vi "DB - [AMS].[Execute].[Message].vi"(0 "connection reference":T3, 1 "DB Connection":T4={"Open"=TRUE, "Close"=TRUE}, 2 "<TOP>":string, 3 "DB - [AMS].[Execute].[Message] Enum":T1, 5 "AMS Execute Message ColNames":T2[](array[typedef])=[enum."[MessageNo]", enum."[SoftwareSolutionId]", enum."[SoftwareSolutionName]", enum."[PlantId]", enum."[MessageLogNo]", enum."[ReceivedOn]", enum."[MessageCode]", enum."[ShortDescription]", enum."[Message]", enum."[SmsMessage]", enum."[TransactionNo]", enum."[TransactionRunNo]", enum."[MessageInitiator]", enum."[Remarks]", enum."[MsgCreatedOn]", enum."[IsToSendSms]", enum."[IsToSendEmail]", enum."[SmsContent]", enum."[EmailContent]", enum."[MobileNos]", enum."[EmailAddresses]"], 9 "<Data> (0xFFFE autodetect)":string[](array[string]), 11 "error in (no error)":errorcluster, 12 "<SIGN>":string, 13 "[MessageNo]":string, 14 "<CONDITIONS>":string) -> (4 "connection reference":T3, 6 "2D data":string[][](array[string]), 10 "SQL Statement":string, 15 "SUMMARY":errorcluster)   [LabVIEW 2013]
uses:
  <vilib>/addons/database/Connection.llb/Conn ObjectReference.ctl
  Controls/DB - OpenClose.ctl
  Controls/DB - [AMS].[Execute].[Message] ColNames.ctl
  Controls/DB - [AMS].[Execute].[Message] Enum.ctl
  Controls/Global AMS.vi
  Controls/Global SRTRS.vi
  <vilib>/addons/database/Connection.llb/DB Tools Open Connec (String).vi
  <vilib>/addons/database/Connection.llb/Conn Execute.vi
  <vilib>/addons/database/Recordset.llb/Rec Fetch Recordset Data (R).vi
  <vilib>/addons/database/Recordset.llb/Rec Destroy - Connection.vi
  <vilib>/addons/database/_DB Variant To Data/Database Variant To Data.xnode
  <vilib>/addons/database/NI_Database_API.lvlib
panel:
  out "Close":errorcluster
  in  "AMS.Execute.MESSAGE (IMPT to leave it in CAPS)":string="AMS.Execute.MESSAGE"
  out "Connection Information":T5={"Connection "="SQL Server 32bit HPEnvy", "Username"="admin", "Password"="admin123"}
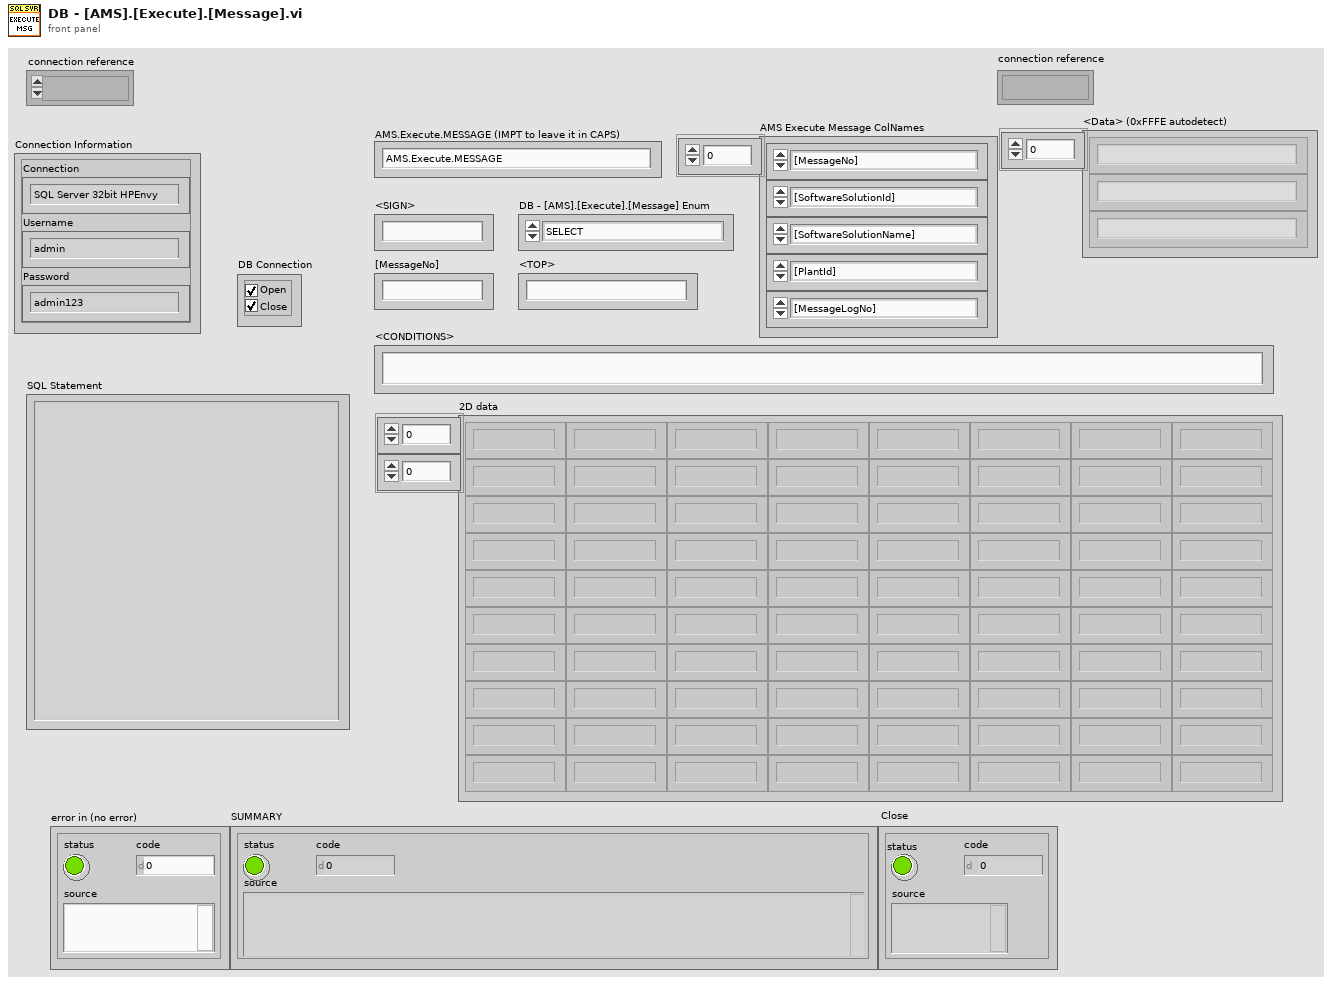
[diagram p1: front panel]
types:
  T1 = typedef "DB - [AMS].[Execute].[Message] Enum.ctl" = enum16{"SELECT", "SELECT (Multi-Conditions)", "UPDATE", "RE-INSERT"}
  T2 = typedef "DB - [AMS].[Execute].[Message] ColNames.ctl" = enum16{"[MessageNo]", "[LanguageId]", "[SoftwareSolutionId]", "[SoftwareSolutionName]", "[PlantId]", "[SystemId]", "[StationId]", "[MessageLogNo]", "[ReceivedOn]", "[MessageCode]", "[ShortDescription]", "[Message]", "[SmsMessage]", "[SuppMessage1]", "[SuppMessage2]", "[SuppMessage3]", "[TransactionNo]", "[TransactionRunNo]", "[MessageInitiator]", "[Remarks]", "[MsgCreatedOn]", "[IsToSendSms]", "[IsToSendEmail]", "[IsToSendCommMedium1]", "[IsToSendCommMedium2]", "[SmsContent]", "[EmailContent]", "[CommMed1Content]", "[CommMed2Content]", "[MobileNos]", "[EmailAddresses]", "[CommMedium1Ids]", "[CommMedium2Ids]", "[LastAttemptedCommMed]", "[LastAttemptedNo]", "[LastAttemptedOn]", "[IsSmsSent]", "[IsEmailSent]", "[IsCommMedium1Sent]", "[IsCommMedium2Sent]", "[OverallSentStatus]", "[StatusUpdatedOn]", "[IsArchived]"}
  T3 = typedef "NI_Database_API.lvlib/Conn ObjectReference.ctl" = refnum<k1>
  T4 = typedef "DB - OpenClose.ctl" = cluster{"Open":bool, "Close":bool}
  T5 = cluster{"Connection ":string, "Username":string, "Password":string}
  T6 = typedef "Enum - InteractiveMode-SubVIMode.ctl" = enum16{"Interactive", "subVI Mode"}
  T7 = typedef "Connection Information Cluster.ctl" = cluster{"Connection ":string, "Username":string, "Password":string}
  T8 = typedef "DB - DB.Schema.Table.ctl" = cluster{"DB":string, "Schema":string, "Table":string}
  T9 = typedef "NI_Database_API.lvlib/Rec ObjectReference.ctl" = refnum<k1>
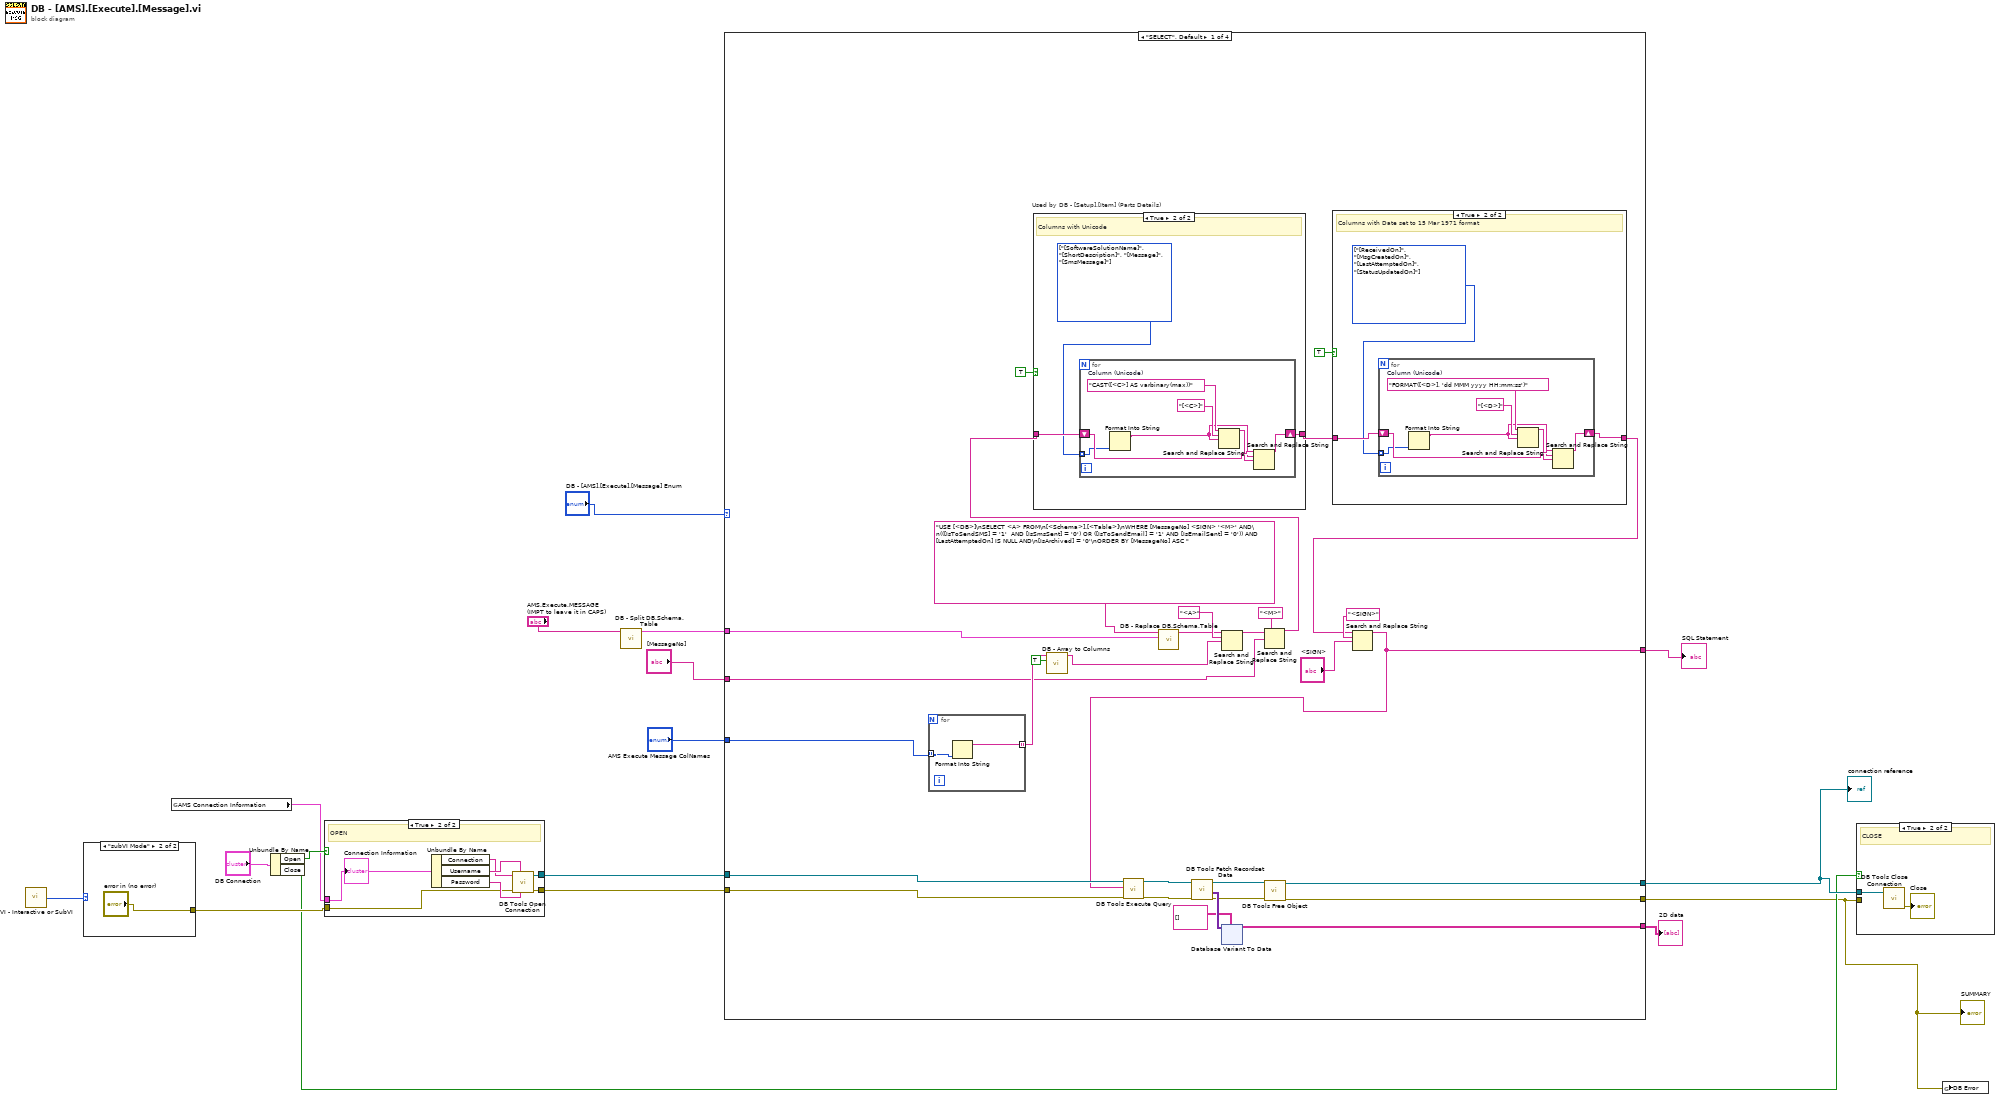
[diagram p0: block diagram]
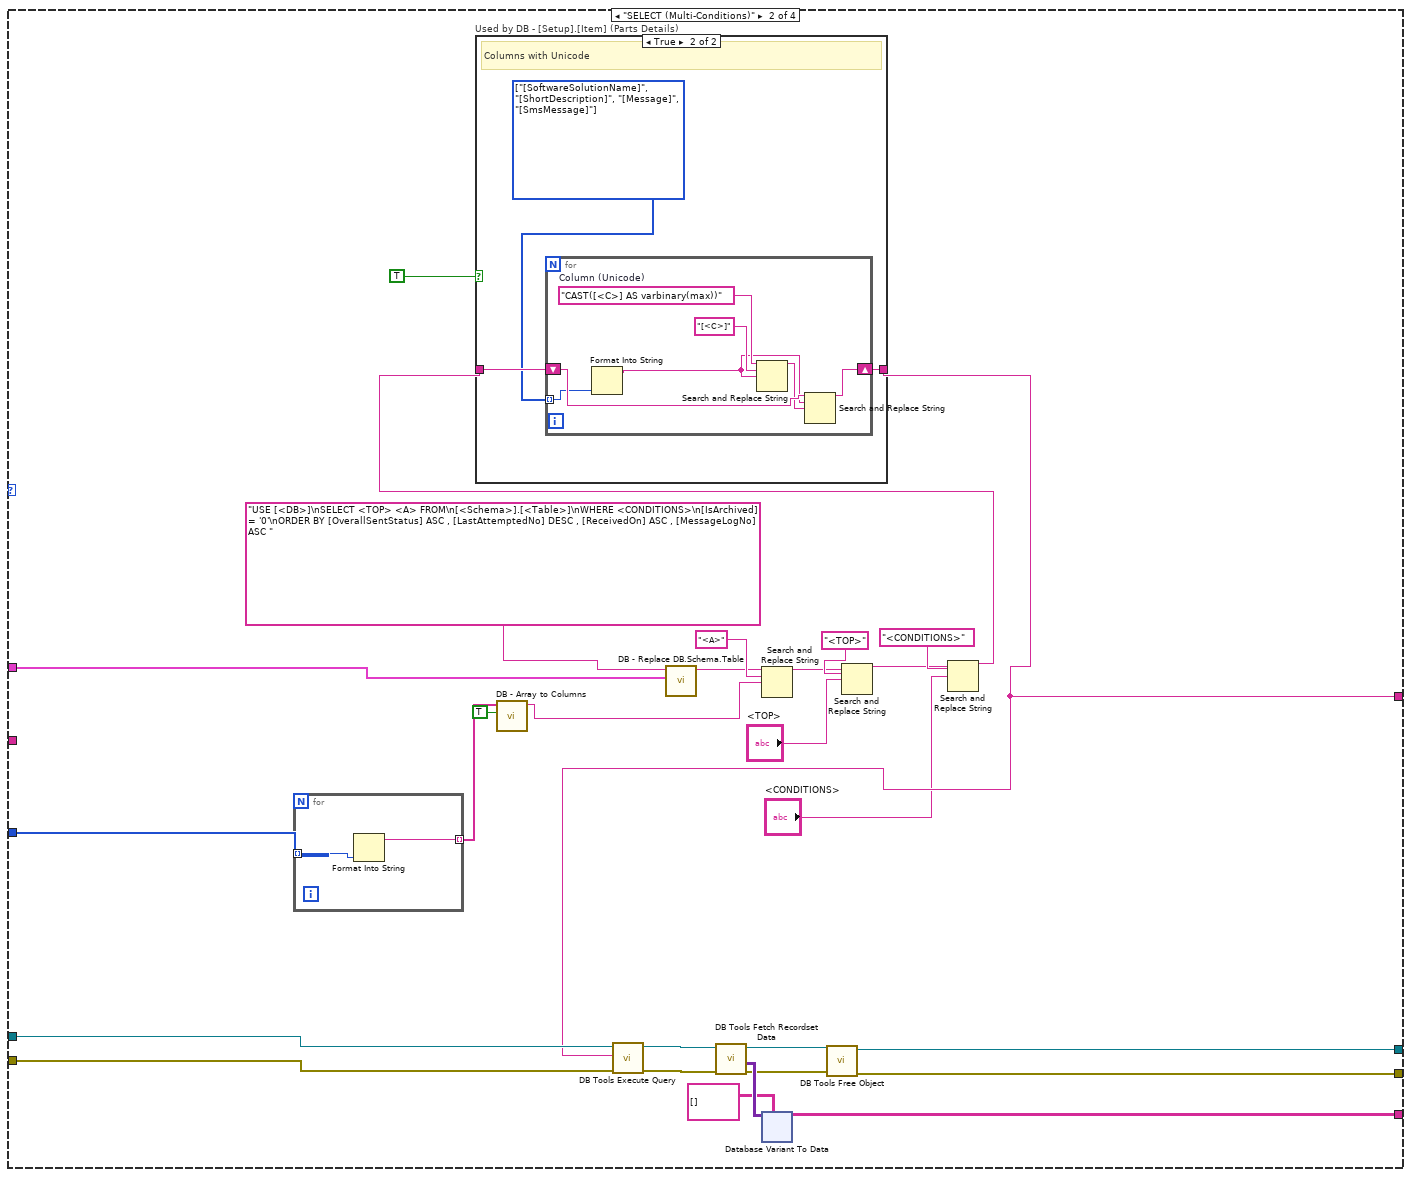
[diagram p4: hidden frame]
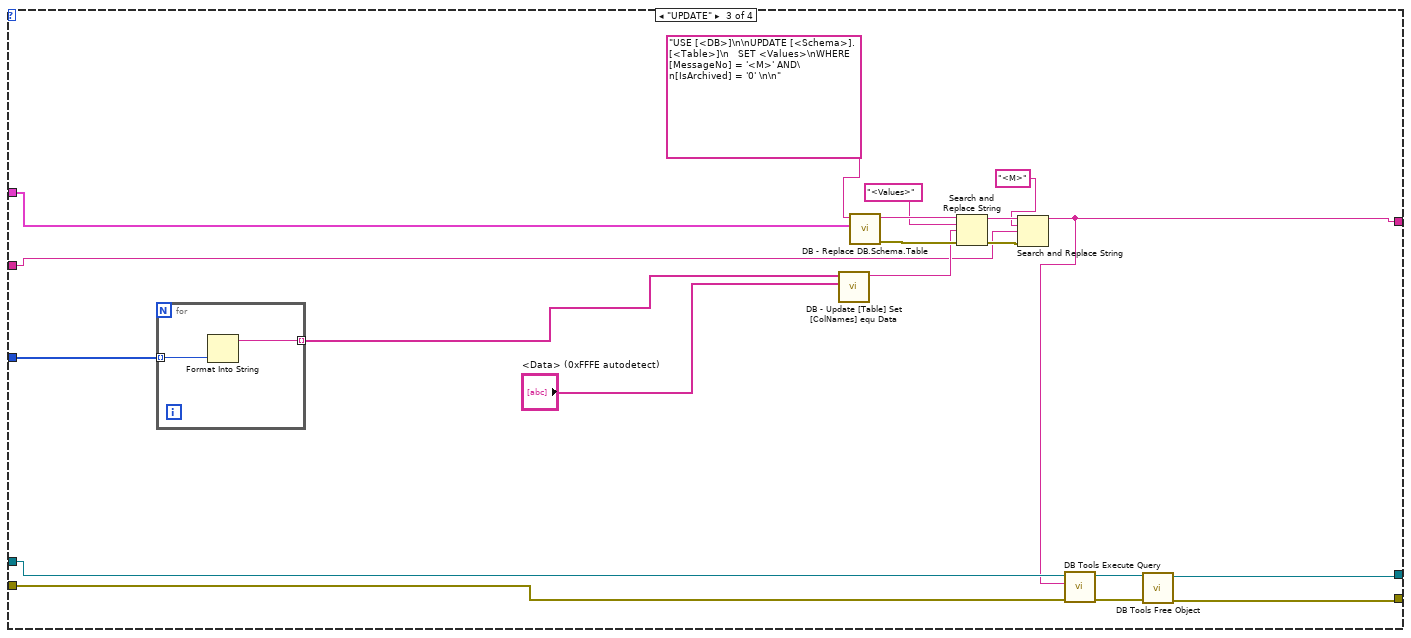
[diagram p6: hidden frame]
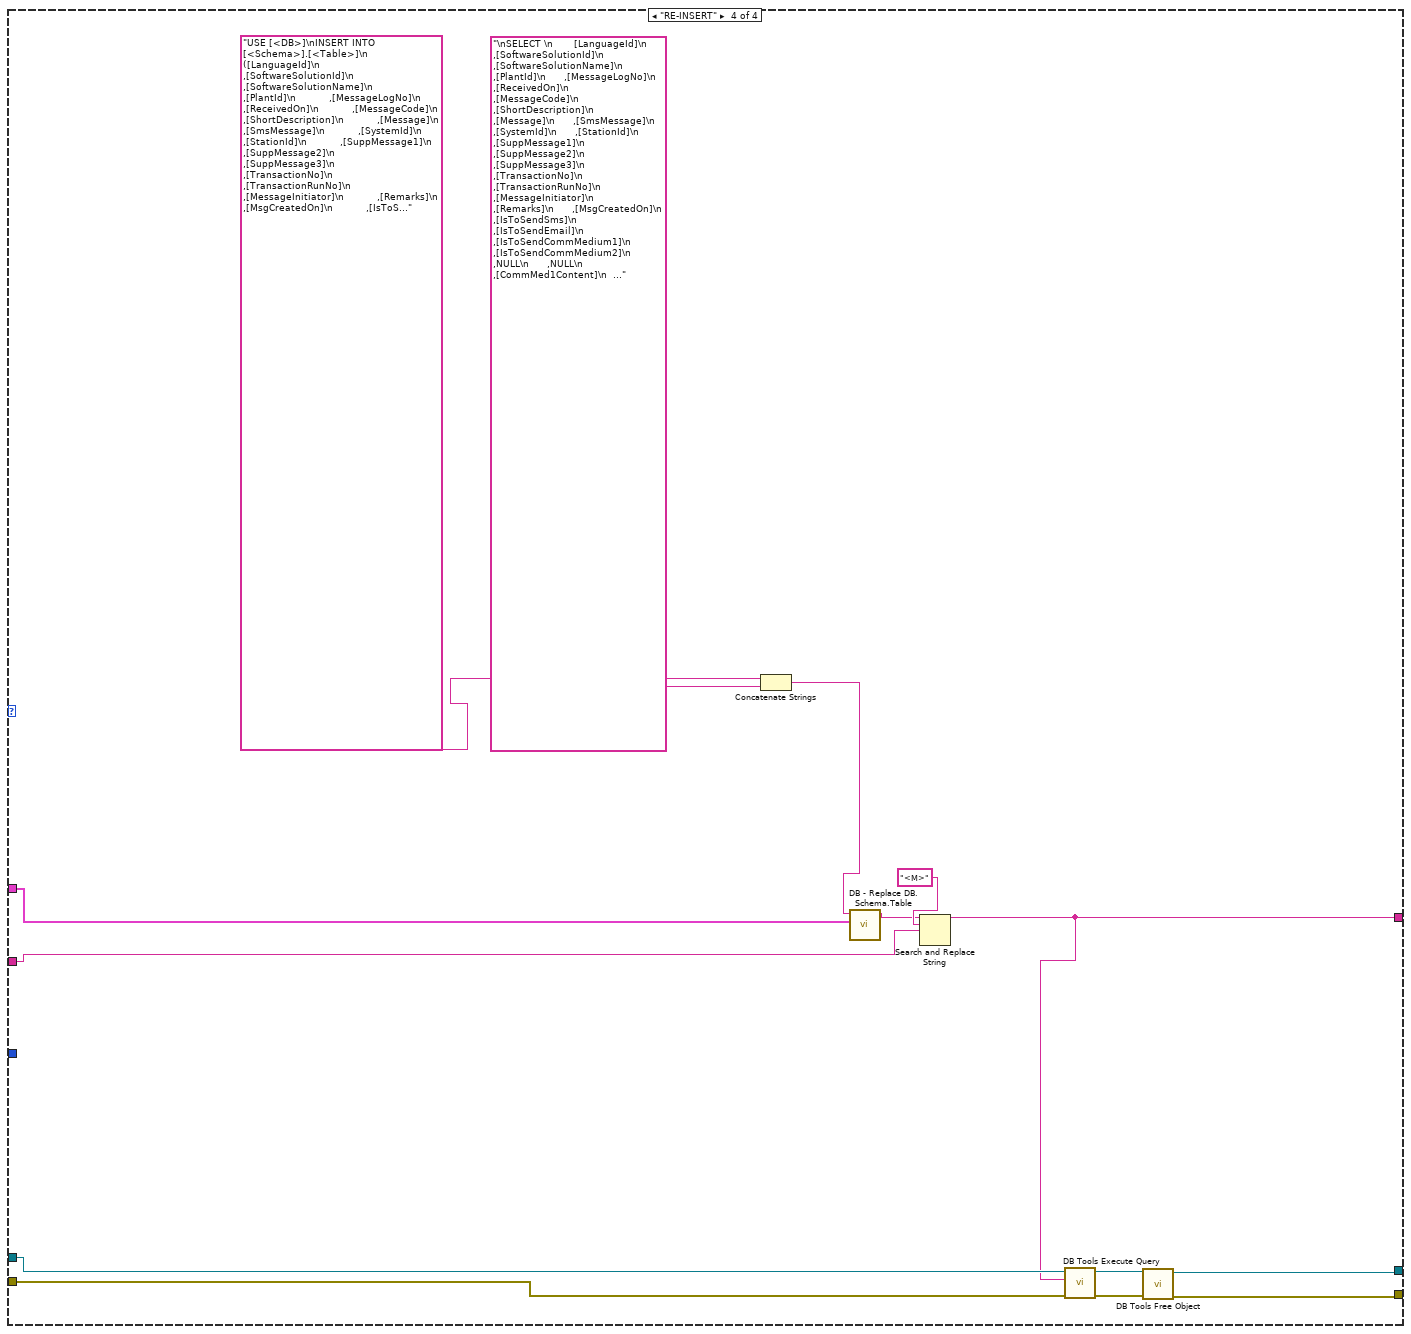
[diagram p7: hidden frame]
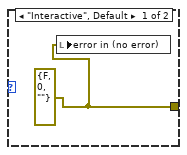
[diagram p9: hidden frame]
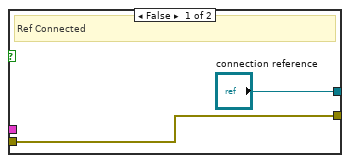
[diagram p10: hidden frame]
diagram:
  n1 = call "VI - Interactive or SubVI.vi"() -> ("Mode"=w15:T6)  [unwired: 5 in]
  n2 = case shown="\"subVI Mode\"" w15 {
    tunnel: [w18 "error in (no error)"] -> w14
    frame "Interactive", Default {
      w18 = errorcluster {"status"=FALSE, "code"=0, "source"=""} ("error in (no error)")
      n3 = local write "error in (no error)"(w18) -> ()
    }
    frame "subVI Mode" {
    }
  }
  n4 = global read "Global AMS.vi" "AMS Connection Information"() -> (w6:T7)
  n5 = Unbundle By Name("DB Connection") -> ("Open"=w16:bool, "Close"=w10:bool)
  n6 = case shown="True" w16 {
    tunnel: ["connection reference" w25] -> w13
    tunnel: w14 -> [w20 w24]
    tunnel: [w20 w23] -> w12
    tunnel: w6 -> [_ w22]
    frame False {
      # "Ref Connected"
    }
    frame True {
      # "OPEN"
      n7 = Unbundle By Name(w22) -> ("Connection"=w27:string, "Username"=w28:string, "Password"=w26:string)
      n8 = call-poly <vilib>:"DB Tools Open Connection.vi"("password"=w26, "userID"=w28, "error in (no error)"=w24, "connection information"=w27) -> ("error out"=w23:errorcluster, "connection reference"=w25:T3)  [unwired: 4 in]
      "Connection Information" <- w22
    }
  }
  n9 = call "DB - Split DB.Schema.Table.vi"("DB.Schema.Table"="AMS.Execute.MESSAGE (IMPT to leave it in CAPS)") -> ("DB.Schema.Table"=w9:T8)  [unwired: 10 in]
  n10 = case shown="\"SELECT\", Default" "DB - [AMS].[Execute].[Message] Enum" {
    tunnel: w13 -> [w52 w148 w215 w239]
    tunnel: w12 -> [w51 w147 w216 w240]
    tunnel: [w50 w146 w218 w242] -> w11
    tunnel: w9 -> [w49 w145 w224 w246]
    tunnel: [w47 w143 w217 w241] -> w8
    tunnel: "AMS Execute Message ColNames" -> [w44 w141 w213 _]
    tunnel: "[MessageNo]" -> [w39 _ w222 w245]
    tunnel: [w36 w133 w214 w238] -> w3
    tunnel: [w32 w132 _ _] -> w1
    frame "SELECT", Default {
      n11 = for {
        tunnel: w44 -> [w82] mode=indexing
        tunnel: [w81] -> w43 mode=indexing
        n12 = Format Into String(w82) -> (resulting string=w81:string)  [unwired: 3 in, 1 out]
      }
      n13 = call "DB - Array to Columns.vi"("Exclude []"=TRUE, "Array"=w43) -> ("[Columns]"=w38:string)  [unwired: 9 in]
      n14 = call "DB - Replace DB.Schema.Table.vi"("DB.Schema.Table"=w49, "string in"="USE [<DB>]\nSELECT <A> FROM\n[<Schema>].[<Table>]\nWHERE [MessageNo] <SIGN> '<M>' AND\n(([IsToSendSMS] = '1'  AND [IsSmsSent] = '0') OR ([IsToSendEmail] = '1' AND [IsEmailSent] = '0')) AND [LastAttemptedOn] IS NULL AND\n[IsArchived] = '0'\nORDER BY [MessageNo] ASC ") -> ("string out"=w33:string)  [unwired: 8 in, 1 out]
      n15 = Search and Replace String(input string=w33, search string="<A>", replace string=w38) -> (result string=w46:string)  [unwired: 5 in, 3 out]
      n16 = Search and Replace String(input string=w46, search string="<M>", replace string=w39) -> (result string=w42:string)  [unwired: 5 in, 3 out]
      n17 = case "Used by DB - [Setup].[Item] (Parts Details)" shown="True" TRUE {
        tunnel: w42 -> [w70 w73]
        tunnel: [w70 w72] -> w30
        frame False {
        }
        frame True {
          w71 = T2[] [enum."[SoftwareSolutionName]", enum."[ShortDescription]", enum."[Message]", enum."[SmsMessage]"] items=["[MessageNo]", "[LanguageId]", "[SoftwareSolutionId]", "[SoftwareSolutionName]", "[PlantId]", "[SystemId]", "[StationId]", "[MessageLogNo]", "[ReceivedOn]", "[MessageCode]", "[ShortDescription]", "[Message]", "[SmsMessage]", "[SuppMessage1]", "[SuppMessage2]", "[SuppMessage3]", "[TransactionNo]", "[TransactionRunNo]", "[MessageInitiator]", "[Remarks]", "[MsgCreatedOn]", "[IsToSendSms]", "[IsToSendEmail]", "[IsToSendCommMedium1]", "[IsToSendCommMedium2]", "[SmsContent]", "[EmailContent]", "[CommMed1Content]", "[CommMed2Content]", "[MobileNos]", "[EmailAddresses]", "[CommMedium1Ids]", "[CommMedium2Ids]", "[LastAttemptedCommMed]", "[LastAttemptedNo]", "[LastAttemptedOn]", "[IsSmsSent]", "[IsEmailSent]", "[IsCommMedium1Sent]", "[IsCommMedium2Sent]", "[OverallSentStatus]", "[StatusUpdatedOn]", "[IsArchived]"]
          # "Columns with Unicode"
          n18 = for {
            shift-right: [w76] -> w72
            shift-left: w73 -> [w80]
            tunnel: w71 -> [w75] mode=indexing
            w79 = "CAST([<C>] AS varbinary(max))"  # Column (Unicode)
            n19 = Format Into String(w75) -> (resulting string=w74:string)  [unwired: 3 in, 1 out]
            n20 = Search and Replace String(input string=w79, search string="[<C>]", replace string=w74) -> (result string=w77:string)  [unwired: 5 in, 3 out]
            n21 = Search and Replace String(input string=w80, search string=w74, replace string=w77) -> (result string=w76:string)  [unwired: 5 in, 3 out]
          }
        }
      }
      n22 = case shown="True" TRUE {
        tunnel: w30 -> [w59 w62]
        tunnel: [w59 w60] -> w29
        frame False {
        }
        frame True {
          w61 = T2[] [enum."[ReceivedOn]", enum."[MsgCreatedOn]", enum."[LastAttemptedOn]", enum."[StatusUpdatedOn]"] items=["[MessageNo]", "[LanguageId]", "[SoftwareSolutionId]", "[SoftwareSolutionName]", "[PlantId]", "[SystemId]", "[StationId]", "[MessageLogNo]", "[ReceivedOn]", "[MessageCode]", "[ShortDescription]", "[Message]", "[SmsMessage]", "[SuppMessage1]", "[SuppMessage2]", "[SuppMessage3]", "[TransactionNo]", "[TransactionRunNo]", "[MessageInitiator]", "[Remarks]", "[MsgCreatedOn]", "[IsToSendSms]", "[IsToSendEmail]", "[IsToSendCommMedium1]", "[IsToSendCommMedium2]", "[SmsContent]", "[EmailContent]", "[CommMed1Content]", "[CommMed2Content]", "[MobileNos]", "[EmailAddresses]", "[CommMedium1Ids]", "[CommMedium2Ids]", "[LastAttemptedCommMed]", "[LastAttemptedNo]", "[LastAttemptedOn]", "[IsSmsSent]", "[IsEmailSent]", "[IsCommMedium1Sent]", "[IsCommMedium2Sent]", "[OverallSentStatus]", "[StatusUpdatedOn]", "[IsArchived]"]
          # "Columns with Date set to 15 Mar 1971 format"
          n23 = for {
            shift-right: [w65] -> w60
            shift-left: w62 -> [w69]
            tunnel: w61 -> [w64] mode=indexing
            w68 = "FORMAT([<D>], 'dd MMM yyyy HH:mm:ss')"  # Column (Unicode)
            n24 = Format Into String(w64) -> (resulting string=w63:string)  [unwired: 3 in, 1 out]
            n25 = Search and Replace String(input string=w68, search string="[<D>]", replace string=w63) -> (result string=w66:string)  [unwired: 5 in, 3 out]
            n26 = Search and Replace String(input string=w69, search string=w63, replace string=w66) -> (result string=w65:string)  [unwired: 5 in, 3 out]
          }
        }
      }
      n27 = Search and Replace String(input string=w29, search string="<SIGN>", replace string="<SIGN>") -> (result string=w36:string)  [unwired: 5 in, 3 out]
      n28 = call-poly <vilib>:"DB Tools Execute Query.vi"("error in (no error)"=w51, "SQL query"=w36, "connection reference"=w52) -> ("error out"=w58:errorcluster, "recordset reference"=w57:T9)  [unwired: 5 in]
      n29 = call-poly <vilib>:"DB Tools Fetch Recordset Data.vi"("error in (no error)"=w58, "recordset reference"=w57) -> ("error out"=w53:errorcluster, "recordset data"=w56:variant[][], "recordset reference out"=w54:T9)  [unwired: 3 in]
      n30 = xnode "Database Variant To Data"("database variant"=w56, "type"=string[][] []) -> ("data"=w32:string[][])  [unwired: 1 in, 1 out]
      n31 = call-poly <vilib>:"DB Tools Free Object.vi"("error in (no error)"=w53, "recordset reference"=w54) -> ("error out"=w47:errorcluster, "connection reference"=w50:T3)  [unwired: 8 in]
    }
    frame "SELECT (Multi-Conditions)" {
      n32 = for {
        tunnel: w141 -> [w167] mode=indexing
        tunnel: [w166] -> w140 mode=indexing
        n33 = Format Into String(w167) -> (resulting string=w166:string)  [unwired: 3 in, 1 out]
      }
      n34 = call "DB - Array to Columns.vi"("Exclude []"=TRUE, "Array"=w140) -> ("[Columns]"=w136:string)  [unwired: 9 in]
      n35 = call "DB - Replace DB.Schema.Table.vi"("DB.Schema.Table"=w145, "string in"="USE [<DB>]\nSELECT <TOP> <A> FROM\n[<Schema>].[<Table>]\nWHERE <CONDITIONS>\n[IsArchived] = '0'\nORDER BY [OverallSentStatus] ASC , [LastAttemptedNo] DESC , [ReceivedOn] ASC , [MessageLogNo] ASC ") -> ("string out"=w134:string)  [unwired: 8 in, 1 out]
      n36 = Search and Replace String(input string=w134, search string="<A>", replace string=w136) -> (result string=w130:string)  [unwired: 5 in, 3 out]
      n37 = Search and Replace String(input string=w130, search string="<TOP>", replace string="<TOP>") -> (result string=w127:string)  [unwired: 5 in, 3 out]
      n38 = Search and Replace String(input string=w127, search string="<CONDITIONS>", replace string="<CONDITIONS>") -> (result string=w139:string)  [unwired: 5 in, 3 out]
      n39 = case "Used by DB - [Setup].[Item] (Parts Details)" shown="True" TRUE {
        tunnel: w139 -> [w155 w158]
        tunnel: [w155 w157] -> w133
        frame False {
        }
        frame True {
          w156 = T2[] [enum."[SoftwareSolutionName]", enum."[ShortDescription]", enum."[Message]", enum."[SmsMessage]"] items=["[MessageNo]", "[LanguageId]", "[SoftwareSolutionId]", "[SoftwareSolutionName]", "[PlantId]", "[SystemId]", "[StationId]", "[MessageLogNo]", "[ReceivedOn]", "[MessageCode]", "[ShortDescription]", "[Message]", "[SmsMessage]", "[SuppMessage1]", "[SuppMessage2]", "[SuppMessage3]", "[TransactionNo]", "[TransactionRunNo]", "[MessageInitiator]", "[Remarks]", "[MsgCreatedOn]", "[IsToSendSms]", "[IsToSendEmail]", "[IsToSendCommMedium1]", "[IsToSendCommMedium2]", "[SmsContent]", "[EmailContent]", "[CommMed1Content]", "[CommMed2Content]", "[MobileNos]", "[EmailAddresses]", "[CommMedium1Ids]", "[CommMedium2Ids]", "[LastAttemptedCommMed]", "[LastAttemptedNo]", "[LastAttemptedOn]", "[IsSmsSent]", "[IsEmailSent]", "[IsCommMedium1Sent]", "[IsCommMedium2Sent]", "[OverallSentStatus]", "[StatusUpdatedOn]", "[IsArchived]"]
          # "Columns with Unicode"
          n40 = for {
            shift-right: [w161] -> w157
            shift-left: w158 -> [w165]
            tunnel: w156 -> [w160] mode=indexing
            w164 = "CAST([<C>] AS varbinary(max))"  # Column (Unicode)
            n41 = Format Into String(w160) -> (resulting string=w159:string)  [unwired: 3 in, 1 out]
            n42 = Search and Replace String(input string=w164, search string="[<C>]", replace string=w159) -> (result string=w162:string)  [unwired: 5 in, 3 out]
            n43 = Search and Replace String(input string=w165, search string=w159, replace string=w162) -> (result string=w161:string)  [unwired: 5 in, 3 out]
          }
        }
      }
      n44 = call-poly <vilib>:"DB Tools Execute Query.vi"("error in (no error)"=w147, "SQL query"=w133, "connection reference"=w148) -> ("error out"=w154:errorcluster, "recordset reference"=w153:T9)  [unwired: 5 in]
      n45 = call-poly <vilib>:"DB Tools Fetch Recordset Data.vi"("error in (no error)"=w154, "recordset reference"=w153) -> ("error out"=w149:errorcluster, "recordset data"=w152:variant[][], "recordset reference out"=w150:T9)  [unwired: 3 in]
      n46 = xnode "Database Variant To Data"("database variant"=w152, "type"=string[][] []) -> ("data"=w132:string[][])  [unwired: 1 in, 1 out]
      n47 = call-poly <vilib>:"DB Tools Free Object.vi"("error in (no error)"=w149, "recordset reference"=w150) -> ("error out"=w143:errorcluster, "connection reference"=w146:T3)  [unwired: 8 in]
    }
    frame "UPDATE" {
      n48 = for {
        tunnel: w213 -> [w233] mode=indexing
        tunnel: [w232] -> w212 mode=indexing
        n49 = Format Into String(w233) -> (resulting string=w232:string)  [unwired: 3 in, 1 out]
      }
      n50 = call "DB - Update [Table] Set [ColNames] equ Data.vi"("<Data> (0xFFFE autodetect)"="<Data> (0xFFFE autodetect)", "[ColumnNames]"=w212) -> ("<Values>"=w225:string)  [unwired: 9 in]
      n51 = call "DB - Replace DB.Schema.Table.vi"("DB.Schema.Table"=w224, "string in"="USE [<DB>]\n\nUPDATE [<Schema>].[<Table>]\n   SET <Values>\nWHERE [MessageNo] = '<M>' AND\n[IsArchived] = '0' \n\n") -> ("error out"=w230:errorcluster, "string out"=w231:string)  [unwired: 8 in]
      n52 = Search and Replace String(input string=w231, search string="<Values>", replace string=w225, error in=w230) -> (result string=w228:string, error out=w227:errorcluster)  [unwired: 4 in, 2 out]
      n53 = Search and Replace String(input string=w228, search string="<M>", replace string=w222, error in=w227) -> (result string=w214:string)  [unwired: 4 in, 3 out]
      n54 = call-poly <vilib>:"DB Tools Execute Query.vi"("error in (no error)"=w216, "SQL query"=w214, "connection reference"=w215) -> ("error out"=w219:errorcluster, "recordset reference"=w220:T9)  [unwired: 5 in]
      n55 = call-poly <vilib>:"DB Tools Free Object.vi"("error in (no error)"=w219, "recordset reference"=w220) -> ("error out"=w217:errorcluster, "connection reference"=w218:T3)  [unwired: 8 in]
    }
    frame "RE-INSERT" {
      n56 = Concatenate Strings("USE [<DB>]\nINSERT INTO [<Schema>].[<Table>]\n           ([LanguageId]\n           ,[SoftwareSolutionId]\n           ,[SoftwareSolutionName]\n           ,[PlantId]\n           ,[MessageLogNo]\n           ,[ReceivedOn]\n           ,[MessageCode]\n           ,[ShortDescription]\n           ,[Message]\n           ,[SmsMessage]\n           ,[SystemId]\n           ,[StationId]\n           ,[SuppMessage1]\n           ,[SuppMessage2]\n           ,[SuppMessage3]\n           ,[TransactionNo]\n           ,[TransactionRunNo]\n           ,[MessageInitiator]\n           ,[Remarks]\n           ,[MsgCreatedOn]\n           ,[IsToSendSms]\n           ,[IsToSendEmail]\n           ,[IsToSendCommMedium1]\n           ,[IsToSendCommMedium2]\n           ,[SmsContent]\n           ,[EmailContent]\n           ,[CommMed1Content]\n           ,[CommMed2Content]\n           ,[MobileNos]\n           ,[EmailAddresses]\n           ,[CommMedium1Ids]\n           ,[CommMedium2Ids]\n           ,[LastAttemptedCommMed]\n           ,[LastAttemptedNo]\n           ,[LastAttemptedOn]\n           ,[IsSmsSent]\n           ,[IsEmailSent]\n           ,[IsCommMedium1Sent]\n           ,[IsCommMedium2Sent]\n           ,[OverallSentStatus]\n           ,[StatusUpdatedOn]\n           ,[IsArchived])\n   \n ", "\nSELECT \n       [LanguageId]\n      ,[SoftwareSolutionId]\n      ,[SoftwareSolutionName]\n      ,[PlantId]\n      ,[MessageLogNo]\n      ,[ReceivedOn]\n      ,[MessageCode]\n      ,[ShortDescription]\n      ,[Message]\n      ,[SmsMessage]\n      ,[SystemId]\n      ,[StationId]\n      ,[SuppMessage1]\n      ,[SuppMessage2]\n      ,[SuppMessage3]\n      ,[TransactionNo]\n      ,[TransactionRunNo]\n      ,[MessageInitiator]\n      ,[Remarks]\n      ,[MsgCreatedOn]\n      ,[IsToSendSms]\n      ,[IsToSendEmail]\n      ,[IsToSendCommMedium1]\n      ,[IsToSendCommMedium2]\n      ,NULL\n      ,NULL\n      ,[CommMed1Content]\n      ,[CommMed2Content]\n      ,[MobileNos]\n      ,[EmailAddresses]\n      ,[CommMedium1Ids]\n      ,[CommMedium2Ids]\n      ,NULL\n      ,NULL\n      ,NULL\n      ,'0'\n      ,'0'\n      ,'0'\n      ,'0'\n      ,'0' \n      ,NULL \n      ,'0' \n\n  FROM [<Schema>].[<Table>]\n WHERE [MessageNo] = '<M>'") -> (w234:string)
      n57 = call "DB - Replace DB.Schema.Table.vi"("DB.Schema.Table"=w246, "string in"=w234) -> ("string out"=w237:string)  [unwired: 8 in, 1 out]
      n58 = Search and Replace String(input string=w237, search string="<M>", replace string=w245) -> (result string=w238:string)  [unwired: 5 in, 3 out]
      n59 = call-poly <vilib>:"DB Tools Execute Query.vi"("error in (no error)"=w240, "SQL query"=w238, "connection reference"=w239) -> ("error out"=w243:errorcluster, "recordset reference"=w244:T9)  [unwired: 5 in]
      n60 = call-poly <vilib>:"DB Tools Free Object.vi"("error in (no error)"=w243, "recordset reference"=w244) -> ("error out"=w241:errorcluster, "connection reference"=w242:T3)  [unwired: 8 in]
    }
  }
  "SUMMARY" <- w8
  "connection reference" <- w11
  "SQL Statement" <- w3
  "2D data" <- w1
  n61 = case shown="True" w10 {
    tunnel: w11 -> [_ w249]
    tunnel: w8 -> [_ _]
    frame False {
      # "Ref Connected"
    }
    frame True {
      # "CLOSE"
      n62 = call <vilib>:"DB Tools Close Connection.vi"("connection reference"=w249) -> ("error out"=→"Close":errorcluster)  [unwired: 6 in]
    }
  }
  n63 = global write "Global SRTRS.vi" "DB Error"(w8) -> ()
